vi "assemblies_features.vi"() -> ()   [LabVIEW 2019]
uses:
  <userlib>/IoT Devices/_subVIs/HTTPComm.ctl
  <userlib>/Onshape/_SubVI/Cluster.ctl
  <userlib>/Onshape/_SubVI/z did wid and eid.vi
panel:
  out "Array":T1(array[cluster])
  out "Device Out":T2
  out "Comm":T3
  out "error out":errorcluster
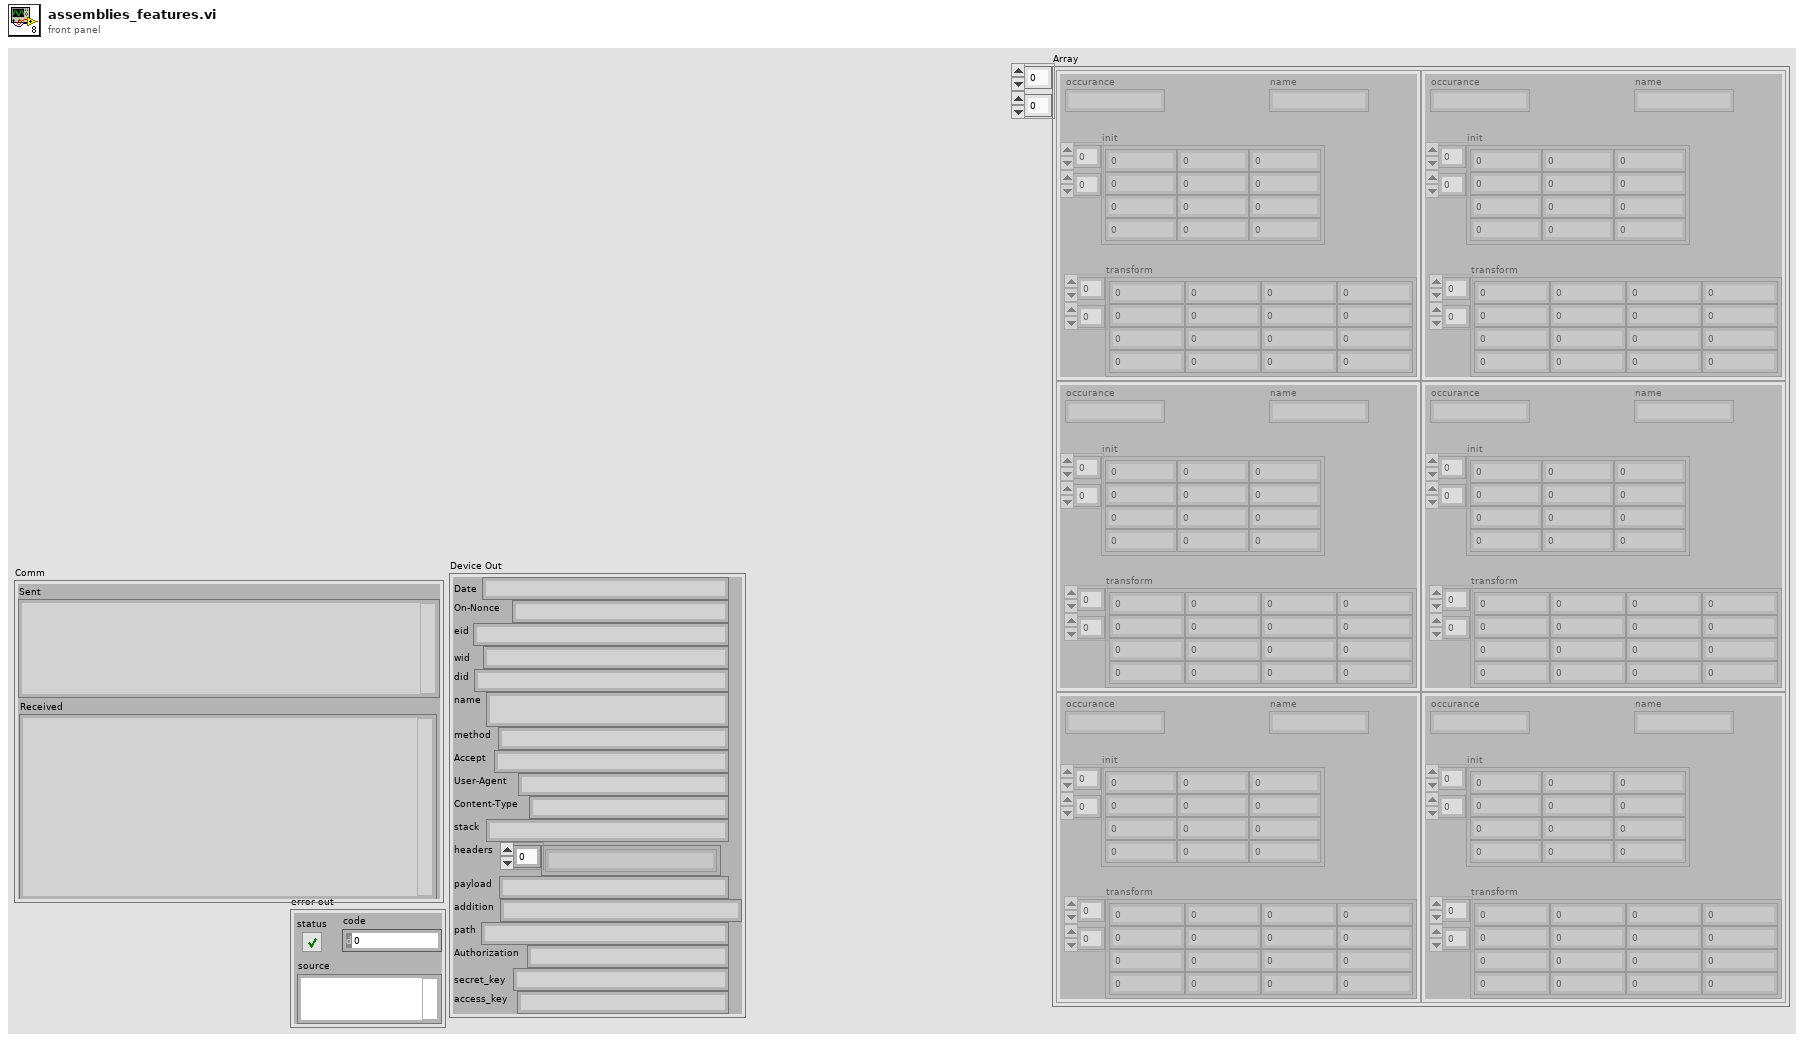
[diagram p1: front panel]
types:
  T1 = cluster{"occurance":string, "init":dbl[][], "transform":dbl[][], "name":string}[][]
  T2 = typedef "Cluster.ctl" = cluster{"Date":string, "On-Nonce":string, "eid":string, "wid":string, "did":string, "name":string, "method":string, "Accept":string, "User-Agent":string, "Content-Type":string, "stack":string, "headers":string[], "payload":string, "addition":string, "path":string, "Authorization":string, "secret_key":string, "access_key":string}
  T3 = typedef "HTTPComm.ctl" = cluster{"url":string, "sent headers":string, "sent body":string, "headers":string, "body":string, "Sent":string, "Received":string}
  T4 = cluster{"rootAssembly":cluster{"elementId":string, "occurrences":cluster{"fixed":bool, "path":string[], "transform":dbl[]}[], "features":cluster{"featureData":cluster{"mateType":string, "matedEntities":cluster{"matedOccurrence":string[], "matedCS":cluster{"origin":dbl[], "xAxis":dbl[], "yAxis":dbl[], "zAxis":dbl[]}}[], "name":string}}[]}}
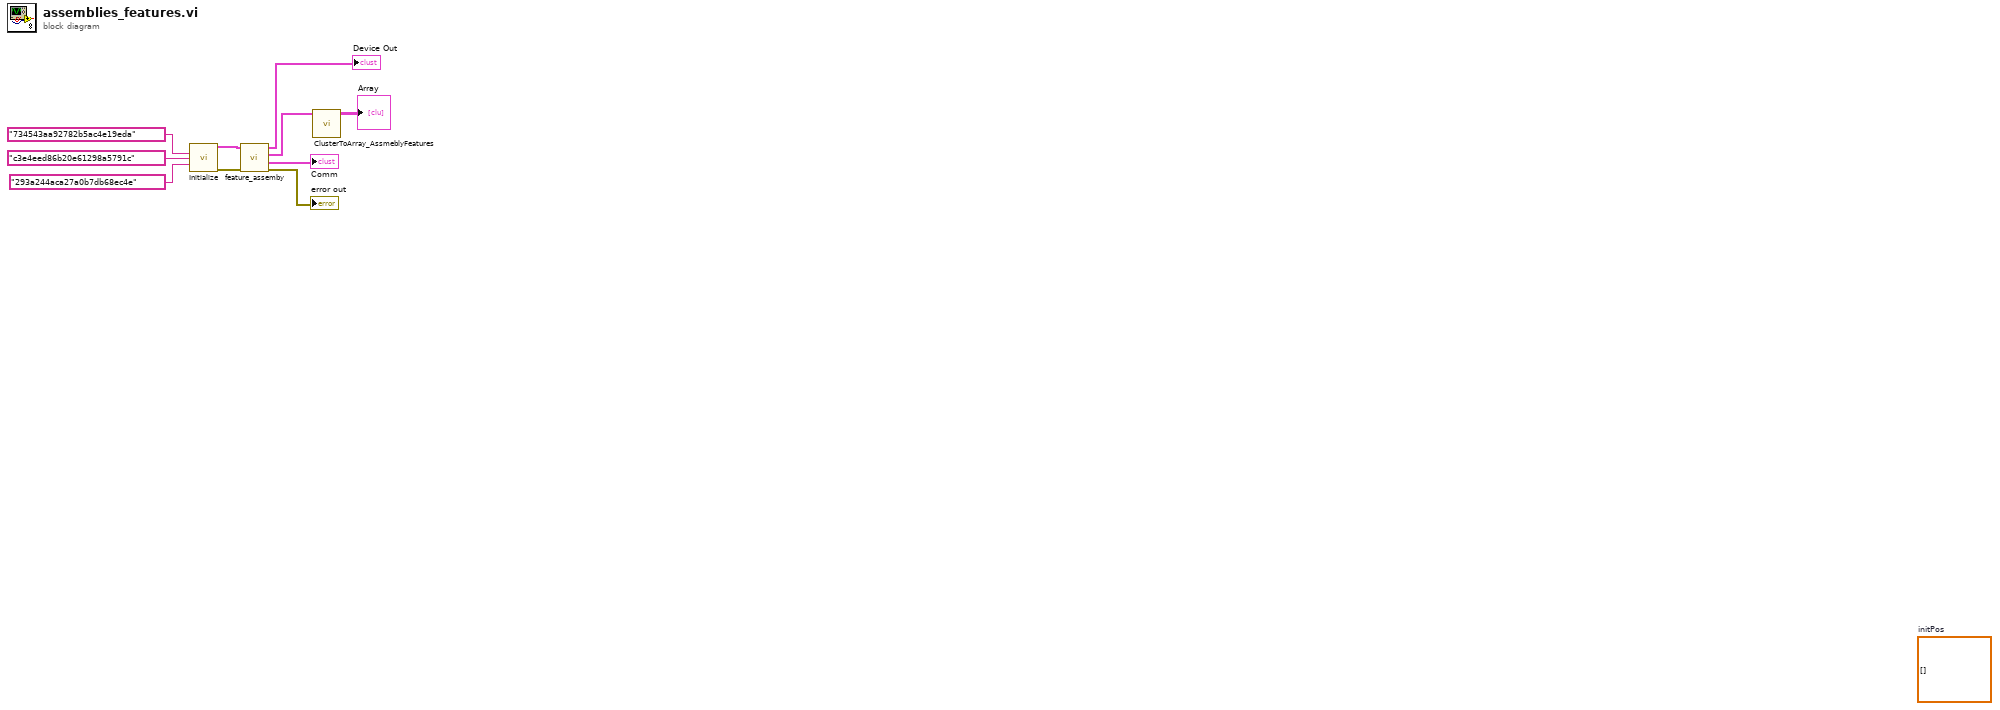
[diagram p0: block diagram]
diagram:
  (unwired) dbl[][] []  # initPos
  n1 = call-poly <userlib>:"Initialize.vi"("did"="734543aa92782b5ac4e19eda", "wid"="c3e4eed86b20e61298a5791c", "eid"="293a244aca27a0b7db68ec4e") -> ("Device Out"=w8:T2, "error out"=w7:errorcluster)  [unwired: 11 in]
  n2 = call <userlib>:"feature_assemby.vi"("error in (no error)"=w7, "Device Out in"=w8) -> ("error out"=→"error out":errorcluster, "Comm"=→"Comm":T3, "value"=w2:T4, "Device Out out"=→"Device Out":T2)  [unwired: 6 in]
  n3 = call <userlib>:"ClusterToArray_AssmeblyFeatures.vi"("value"=w2) -> ("Array"=→"Array":T1)  [unwired: 10 in]
